vi "Data JSON.vi"(8 "error in (no error)":errorcluster, 11 "Identify in":refnum<class "Identify.lvclass">) -> (0 "error out":errorcluster, 2 "Data JSON":string, 3 "Identify out":refnum<class "Identify.lvclass">)   [LabVIEW 2022 SP3, in "obs-websocket-lv.lvlib" / "Identify.lvclass"]
uses:
  Identify.lvclass
  Identify.lvclass/Identify.ctl
  <vilib>/IlluminatedG/lv-web-crypto/lv-json/JSON/JSON.lvlib
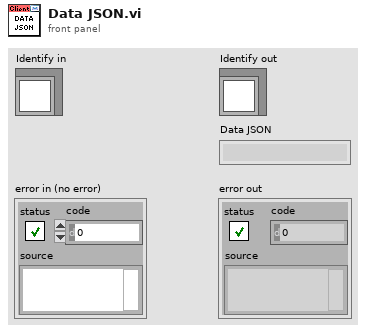
[diagram p1: front panel]
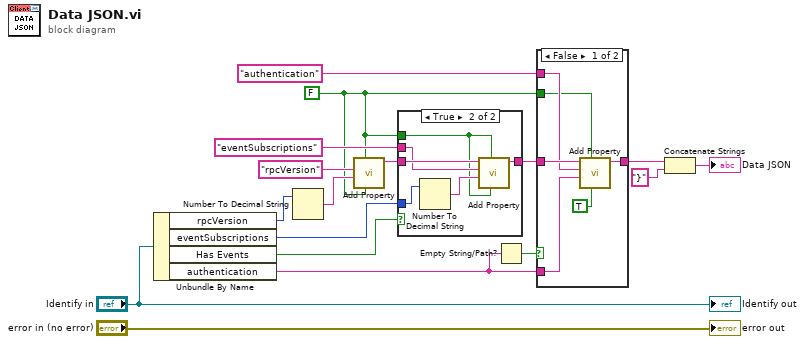
[diagram p0: block diagram]
diagram:
  w1 = FALSE
  n1 = Unbundle By Name("Identify in") -> ("rpcVersion"=w14:i32, "eventSubscriptions"=w10:u32, "Has Events"=w11:bool, "authentication"=w3:string)
  n2 = Number To Decimal String(number=w14) -> (decimal integer string=w13:string)  [unwired: 1 in]
  n3 = call <vilib>:"Add Property.vi"("String?"=w1, "Include Empty?"=w1, "Value"=w13, "Property Name"="rpcVersion") -> ("String out"=w12:string)  [unwired: 7 in]
  n4 = case shown="True" w11 {
    tunnel: w12 -> [w18 w24]
    tunnel: w10 -> [_ w23]
    tunnel: "eventSubscriptions" ("Property Name") -> [_ w21]
    tunnel: [w18 w20] -> w7
    tunnel: w1 -> [_ w19]
    frame False {
    }
    frame True {
      n5 = Number To Decimal String(number=w23) -> (decimal integer string=w22:string)  [unwired: 1 in]
      n6 = call <vilib>:"Add Property.vi"("String?"=w19, "Include Empty?"=w19, "Value"=w22, "Property Name"=w21, "String In"=w24) -> ("String out"=w20:string)  [unwired: 6 in]
    }
  }
  n7 = Empty String/Path?(string/path=w3) -> (empty?=w8:bool)
  n8 = case shown="False" w8 {
    tunnel: w7 -> [w30 w31]
    tunnel: [w28 w31] -> w6
    tunnel: w3 -> [w29 _]
    tunnel: "authentication" ("Property Name") -> [w27 _]
    tunnel: w1 -> [w26 _]
    frame False {
      n9 = call <vilib>:"Add Property.vi"("String?"=TRUE, "Include Empty?"=w26, "Value"=w29, "Property Name"=w27, "String In"=w30) -> ("String out"=w28:string)  [unwired: 6 in]
    }
    frame True {
    }
  }
  n10 = Concatenate Strings(w6, "}" ("string")) -> (→"Data JSON":string)
  "error out" <- "error in (no error)"
  "Identify out" <- "Identify in"
